vi "BLE - Enable notifications.vi"(6 "Conn Status":T1={"MAC Address"="", "cnx handle"=0, "cnx flags"=0, "Address Type"=0, "Connection Interval (ms)"=125, "Timeout(ms)"=125, "Latency"=125, "bonding handle"=0} {"Address Type" items=["Public", "Random"]}, 7 "Descriptor handle":u16, 8 "Error In":errorcluster, 10 "Enable notifications":bool, 11 "COM Bluegiga in":refnum<visa-resource-name>) -> (0 "Error Out":errorcluster, 3 "COM Bluegiga out":refnum<visa-resource-name>)   [LabVIEW 2016]
uses:
  <vilib>/BLE/type_def/connection_status_bundle.ctl
  <vilib>/BLE/type_def/address_type.ctl
  <vilib>/BLE/ble_functions/ble_write_by_handle_uint16.vi
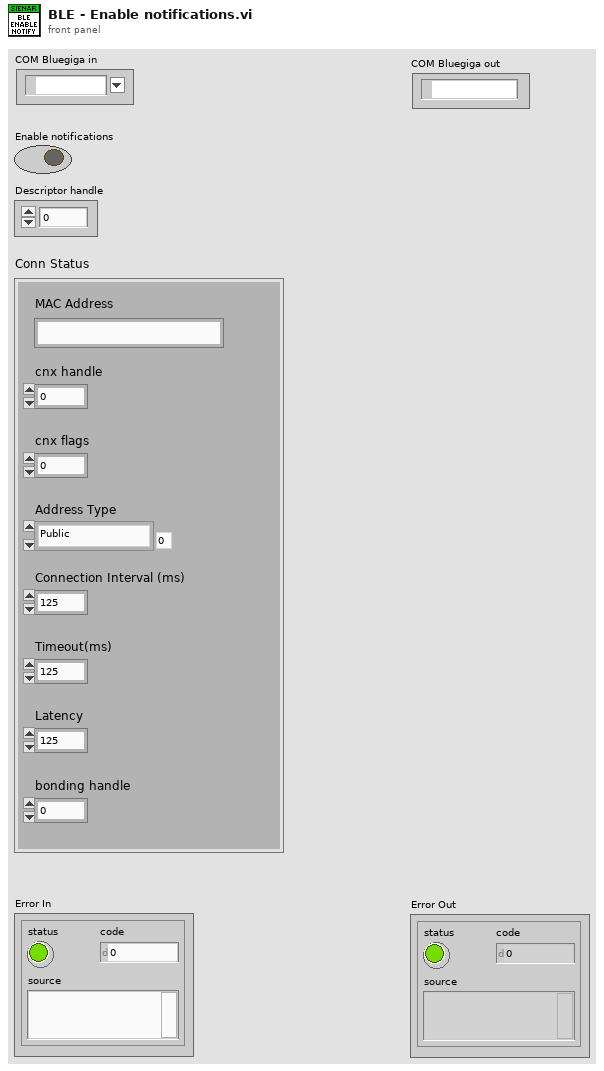
[diagram p1: front panel]
types:
  T1 = typedef "connection_status_bundle.ctl" = cluster{"MAC Address":string, "cnx handle":u8, "cnx flags":u8, "Address Type":T2, "Connection Interval (ms)":u16, "Timeout(ms)":u16, "Latency":u16, "bonding handle":u8}
  T2 = typedef "address_type.ctl" = u8
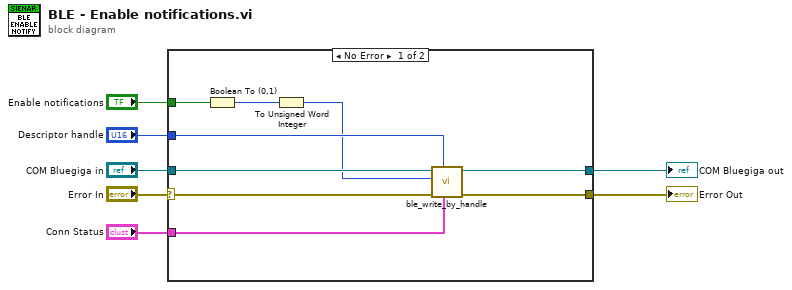
[diagram p0: block diagram]
diagram:
  n1 = case shown="No Error" "Error In" {
    selector: "Error In" -> [w15 w17]
    tunnel: [w14 w17] -> w6
    tunnel: "COM Bluegiga in" -> [w16 w18]
    tunnel: [w13 w18] -> w4
    tunnel: "Descriptor handle" -> [w12 _]
    tunnel: "Conn Status" -> [w11 _]
    tunnel: "Enable notifications" -> [w10 _]
    frame No Error {
      n2 = Boolean To (0,1)(Boolean=w10) -> (0, 1=w9:i16)
      n3 = To Unsigned Word Integer(number=w9) -> (unsigned 16bit integer=w8:u16)
      n4 = call-poly <vilib>:"ble_write_by_handle.vi"("Connection Status"=w11, "Handle"=w12, "error in (no error)"=w15, "Value(uint16)"=w8, "COM Bluegiga in"=w16) -> ("error out"=w14:errorcluster, "COM Bluegiga out"=w13:refnum<visa-resource-name>)  [unwired: 5 in]
    }
    frame Error {
    }
  }
  "Error Out" <- w6
  "COM Bluegiga out" <- w4
